vi "le motv dando certo.vi"() -> ()   [LabVIEW 2016]
uses:
  Program Files (x86)/National Instruments/LabVIEW 2016/examples/Instrument IO/Serial/support/Serial - Settings.ctl
  Program Files (x86)/National Instruments/LabVIEW 2016/examples/Instrument IO/Serial/support/Serial - XON-XOFF Characters.ctl
  Program Files (x86)/National Instruments/LabVIEW 2016/examples/Instrument IO/Serial/support/Serial - ASCII Characters.ctl
  <vilib>/Instr/_visa.llb/VISA Configure Serial Port (Instr).vi
panel:
  out "output waveform":waveform(dbl)(graph)
  out "remaining string":string
  out "error out 2":errorcluster
  out "velocidade":dbl
  out "output 1":dbl
  out "# bytes lidos":u32
  in  "Termination Character":u8=10 format="%.0x"
  in  "End Write on Termination Character?":bool=TRUE
  in  "VISA resource name":refnum<visa-resource-name>="COM1"
  in  "XON/XOFF Characters":T1={"XON"=enum."DC1", "XOFF"=enum."DC3"}
  in  "Serial Settings":T3={"baud rate"=9600, "data bits"=8, "parity"=enum."None", "stop bits"=10, "flow control"=0} {"flow control" items=["None"=0, "XON/XOFF"=1, "RTS/CTS"=2, "DTR/DSR"=4]; "stop bits" items=["1.0"=10, "1.5"=15, "2.0"=20]; "data bits" min=5 max=8 step=1; "baud rate" items=["75"=75, "110"=110, "134"=134, "150"=150, "300"=300, "600"=600, "1200"=1200, "1800"=1800, "2400"=2400, "4800"=4800, "7200"=7200, "9600"=9600, "14400"=14400, "19200"=19200, "28800"=28800, "38400"=38400, "56000"=56000, "57600"=57600, "115200"=115200, "128000"=128000, "230400"=230400]}
  in  "End Read on Termination Character?":bool=TRUE
  out "Response":string
  in  "Read Count":u32=1000
  in  "Command":string="*IDN?"
  in  "Read":bool
  in  "Stop":bool
  in  "Write":bool
  # "SAÍDA DA SCAN FROM STRING"
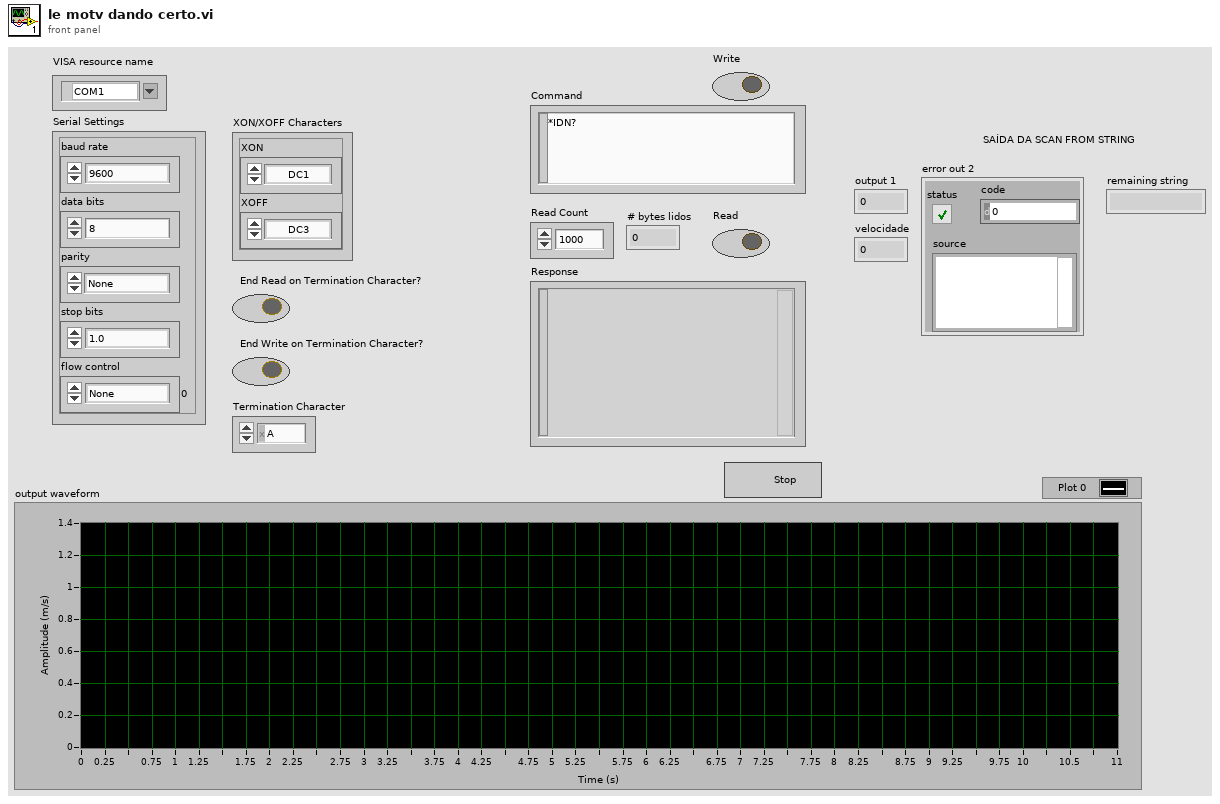
[diagram p1: front panel]
types:
  T1 = typedef "Serial - XON-XOFF Characters.ctl" = cluster{"XON":T2, "XOFF":T2}
  T2 = typedef "Serial - ASCII Characters.ctl" = enum16{"NUL", "SOH", "STX", "ETX", "EOT", "ENQ", "ACK", "BEL", "BS", "HT", "LF", "VT", "FF", "CR", "SO", "SI", "DLE", "DC1", "DC2", "DC3", "DC4", "NAK", "SYN", "ETB", "CAN", "EM", "SUB", "ESC", "FS", "GS", "RS", "US", "SP", "!", "\"", "#", "$", "%", "&", "'", "(", ")", "*", "+", ",", "- (-)", ".", "/", "0", "1", "2", "3", "4", "5", "6", "7", "8", "9", ":", ";", "<", "=", ">", "?", "@", "A", "B", "C", "D", "E", "F", "G", "H", "I", "J", "K", "L", "M", "N", "O", "P", "Q", "R", "S", "T", "U", "V", "W", "X", "Y", "Z", "[", "\\", "]", "^", "_", "`", "a", "b", "c", "d", "e", "f", "g", "h", "i", "j", "k", "l", "m", "n", "o", "p", "q", "r", "s", "t", "u", "v", "w", "x", "y", "z", "{", "|", "}", "~"}
  T3 = typedef "Serial - Settings.ctl" = cluster{"baud rate":u32, "data bits":u16, "parity":enum16{"None", "Odd", "Even", "Mark", "Space"}, "stop bits":u16, "flow control":u16}
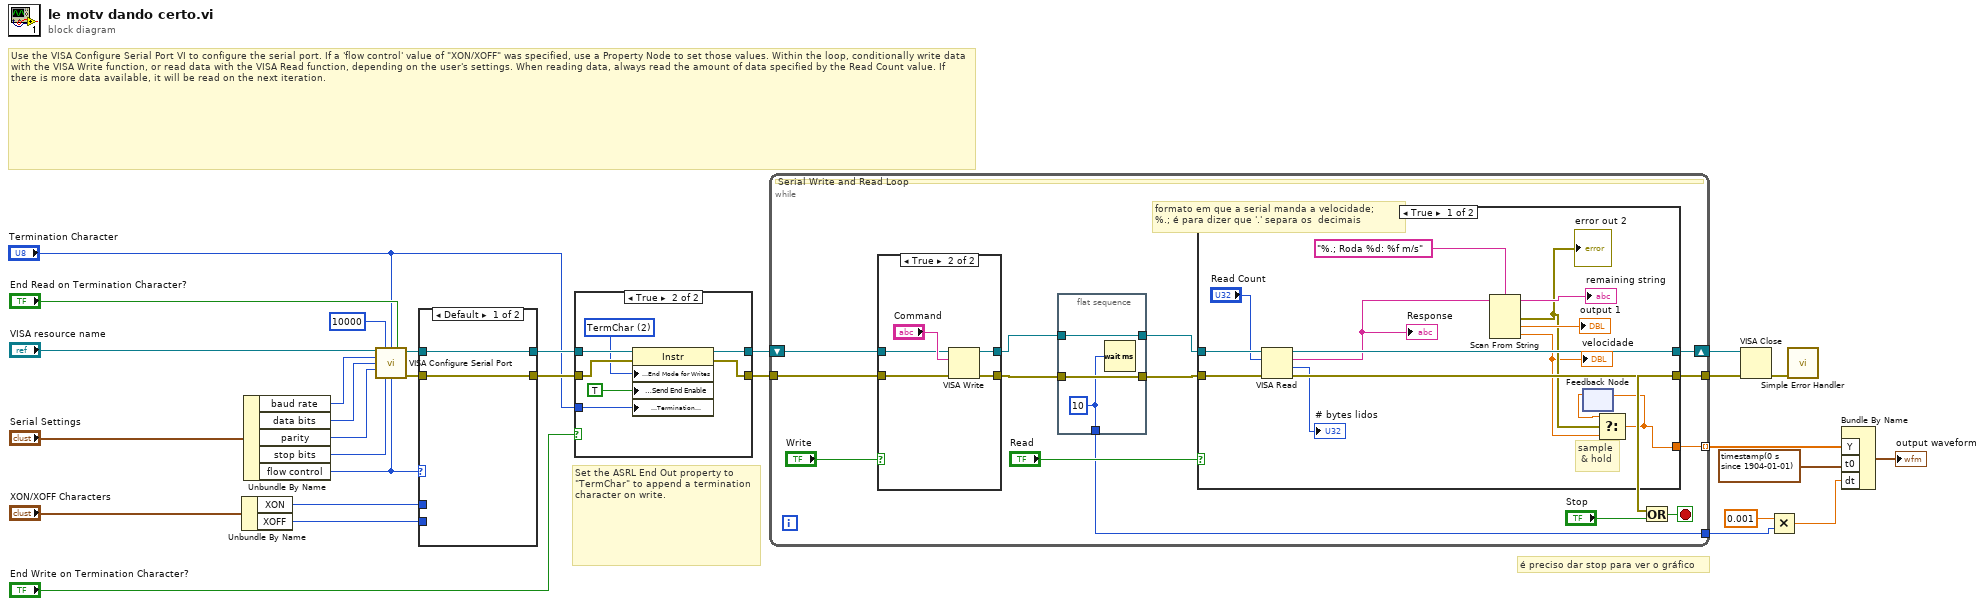
[diagram p0: block diagram]
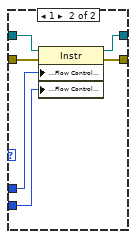
[diagram p3: hidden frame]
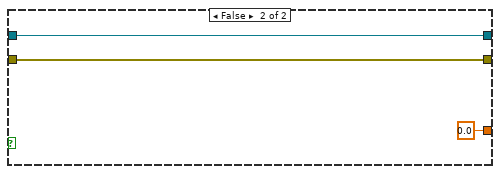
[diagram p5: hidden frame]
diagram:
  # "é preciso dar stop para ver o gráfico"
  # "Set the ASRL End Out property to \"TermChar\" to append a termination character on write."
  # "Use the VISA Configure Serial Port VI to configure the serial port. If a 'flow control' value of \"XON/XOFF\" was specified, use a Property Node to set those values. Within the loop, conditionally write data with the VISA Write function, or read data with the VISA Read function, depending on the user's settings. When reading data, always read the amount of data specified by the Read Count value. If there is more data available, it will be read on the next iteration."
  n1 = Unbundle By Name("XON/XOFF Characters") -> ("XON"=w15:T2, "XOFF"=w14:T2)
  n2 = Unbundle By Name("Serial Settings") -> ("baud rate"=w22:u32, "data bits"=w23:u16, "parity"=w24:enum16{"None", "Odd", "Even", "Mark", "Space"}, "stop bits"=w25:u16, "flow control"=w16:u16)
  n3 = call-poly "VISA Configure Serial Port"("VISA resource name"="VISA resource name", "timeout (10sec)"=u32 10000, "termination char\n(0xA = '\\n' = LF)"="Termination Character", "Enable Termination\nChar (T)"="End Read on Termination Character?", "baud rate (9600)"=w22, "data bits (8)"=w23, "parity (0:none)"=w24, "stop bits (10: 1 bit)"=w25, "flow control (0:none)"=w16) -> ("VISA resource name out"=w26:refnum<visa-resource-name>, "error out"=w27:errorcluster)  [unwired: 1 in, 4 out]
  n4 = case shown="Default" w16 {
    tunnel: [w30 w37] -> w13
    tunnel: [w31 w36] -> w11
    tunnel: w27 -> [w30 w35]
    tunnel: w26 -> [w31 w34]
    tunnel: w15 -> [_ w33]
    tunnel: w14 -> [_ w32]
    frame Default {
    }
    frame 1 {
      n5 = property class="Instr"(reference=w34, error in=w35, "Serial Settings:Flow Control XON Character"=w33, "Serial Settings:Flow Control XOFF Character"=w32) -> (reference out=w36:refnum<visa-resource-name>, error out=w37:errorcluster)
    }
  }
  n6 = case shown="True" "End Write on Termination Character?" {
    tunnel: w11 -> [w38 w46]
    tunnel: w13 -> [w39 w45]
    tunnel: [w38 w44] -> w10
    tunnel: [w39 w43] -> w12
    tunnel: "Termination Character" -> [_ w41]
    frame False {
    }
    frame True {
      w42 = u16 2 items=["None", "LastBit", "TermChar", "Break"] ("Serial Settings:Serial End Mode for Writes")
      n7 = property class="Instr"(reference=w46, error in=w45, "Serial Settings:End Mode for Writes"=w42, "Message Based Settings:Send End Enable"=TRUE, "Message Based Settings:Termination Character"=w41) -> (reference out=w44:refnum<visa-resource-name>, error out=w43:errorcluster)
    }
  }
  n8 = while {
    shift-right: [w60] -> w17
    shift-left: w10 -> [w59]
    tunnel: w12 -> [w58]
    tunnel: [w55] -> w18
    tunnel: [w48] -> w6 mode=indexing
    tunnel: [w47] -> w2
    stop <- w56 stop-if-true
    # "formato em que a serial manda a velocidade;\n%.; é para dizer que '.' separa os  decimais"
    # "Serial Write and Read Loop"
    n9 = case shown="True" "Write" {
      tunnel: w59 -> [w65 w69]
      tunnel: w58 -> [w64 w68]
      tunnel: [w65 w67] -> w52
      tunnel: [w64 w66] -> w49
      frame False {
      }
      frame True {
        n10 = VISA Write(VISA resource name=w69, write buffer="Command", error in (no error)=w68) -> (VISA resource name out=w67:refnum<visa-resource-name>, error out=w66:errorcluster)  [unwired: 1 out]
      }
    }
    n11 = flat-sequence {
      tunnel: [w63] -> w50
      tunnel: w49 -> [w63]
      tunnel: [w62] -> w51
      tunnel: w52 -> [w62]
      tunnel: [w61] -> w47
      frame #0 {
        w61 = u32 10 ("milliseconds to wait")
        n12 = Wait (ms)(milliseconds to wait=w61) -> ()  [unwired: 1 out]
      }
    }
    n13 = case shown="True" "Read" {
      tunnel: [w82 w87] -> w60
      tunnel: w51 -> [w84 w87]
      tunnel: [w80 w86] -> w55
      tunnel: w50 -> [w83 w86]
      tunnel: [w73 0.0 ("velocidade")] -> w48
      frame True {
        # "sample\n & hold"
        n14 = VISA Read(VISA resource name=w84, byte count="Read Count", error in (no error)=w83) -> (VISA resource name out=w82:refnum<visa-resource-name>, read buffer=w75:string, return count=→"# bytes lidos":u32, error out=w80:errorcluster)
        "Response" <- w75
        n15 = Scan From String(format string="%.; Roda %d: %f m/s", input string=w75) -> (remaining string=→"remaining string":string, error out=w74:errorcluster, output 1=→"output 1":dbl, output 2=w71:dbl)  [unwired: 4 in, 1 out]
        "velocidade" <- w71
        "error out 2" <- w74
        n16 = feedback #1() -> (w72:dbl)  [unwired: 1 in]
        n17 = Select(t=w72, s=w74, f=w71) -> (s? t:f=w73:dbl)
        n18 = feedback-in #1(w73) -> ()
      }
      frame False {
      }
    }
    n19 = Or(x=w55, y="Stop") -> (x .or. y?=w56:bool)
  }
  n20 = VISA Close(VISA resource name=w17, error in (no error)=w18) -> (error out=w19:errorcluster)
  n21 = Multiply(x=0.001, y=w2) -> (x*y=w1:dbl)
  n22 = call <vilib>:"Simple Error Handler.vi"("error in (no error)"=w19) -> ()  [unwired: 1 in, 8 out]
  n23 = Bundle By Name("Y"=w6, "t0"=timestamp(0 s since 1904-01-01), "dt"=w1) -> (→"output waveform":waveform(dbl))  [unwired: 1 in]
